vi "uintAddArrayElements.vi"(8 "Error in (no error)":errorcluster, 11 "Uint array in":refnum<class "UintClass.lvclass">[](array[class])) -> (0 "Error out":errorcluster, 1 "Timing":u32, 3 "Sum":refnum<class "UintClass.lvclass">, 5 "Timeout?":bool)   [LabVIEW 2011, in "UintClass.lvclass"]
uses:
  UintClass.lvclass
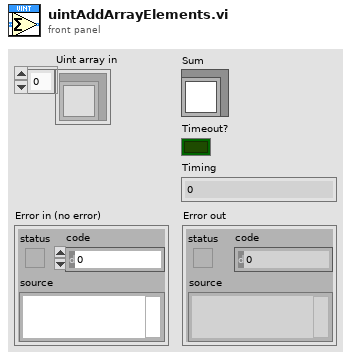
[diagram p1: front panel]
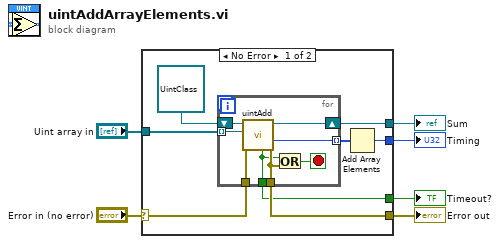
[diagram p0: block diagram]
diagram:
  n1 = case shown="No Error" "Error in (no error)" {
    selector: "Error in (no error)" -> [w12 w23]
    tunnel: "Uint array in" -> [w14 _]
    tunnel: [w11 w23] -> w4
    tunnel: [w10 _] -> w3
    tunnel: [w9 _] -> w2
    tunnel: [w7 _] -> w1
    frame No Error {
      n2 = for {
        tunnel: w14 -> [w22] mode=indexing
        shift-right: [w21] -> w10
        shift-left: refnum<class "UintClass.lvclass"> refnum ("Uint1 + Uint2") -> [w20]
        tunnel: [w18] -> w8 mode=indexing
        tunnel: w12 -> [w17]
        tunnel: [w16] -> w11
        tunnel: [w15] -> w9
        stop <- w19 stop-if-true
        n3 = call "uintAdd.vi"("Error in (no error)"=w17, "Uint2 in"=w22, "Uint1 in"=w20) -> ("Error out"=w16:errorcluster, "Timing"=w18:u32, "Uint1 + Uint2"=w21:refnum<class "UintClass.lvclass">, "Timeout?"=w15:bool)  [unwired: 5 in]
        n4 = Or(x=w15, y=w16) -> (x .or. y?=w19:bool)
      }
      n5 = Add Array Elements(numeric array=w8) -> (sum=w7:u32)
    }
    frame Error {
    }
  }
  "Error out" <- w4
  "Sum" <- w3
  "Timing" <- w1
  "Timeout?" <- w2
